vi "Drive Controller.vi"(8 "error in":errorcluster) -> ()   [LabVIEW 2015]
doc: "This VI executes continuously carrying out the current operation and responding to updates or new operation requests. It will often contain the timing or control code that is difficult to place directly in TeleOp. This VI generally opens all sensors and motors and isolates the rest of the robot code from knowing implementation details of how the operations are carried out."
uses:
  Drive Setpoints.ctl
  Drive Operations.ctl
  <vilib>/Rock Robotics/WPI/SafetyOutput/WPI_SafetyOutputConfigMenu.ctl
  <vilib>/Rock Robotics/WPI/CAN/TalonSRX/WPI_CANTalonSRX_APIControlMode.ctl
  <vilib>/Rock Robotics/WPI/CAN/TalonSRX/WPI_CANTalonSRX_APIFeedbackSelect.ctl
  <vilib>/Rock Robotics/WPI/MotorControl/WPI_MotorControlOpenCANTalonSRX.vi
  <vilib>/Rock Robotics/WPI/RobotDrive/WPI_RobotDriveOpen2MotorWithExistingMotors.vi
  Support Code/navX Library v2/navX Library v2.lvlib
panel:
  out "Setpoints":T1(graph)
  out "Current\nCmd":string
  # "Tip: It may be helpful to observe inputs and sensor values.\nYou may also want to display tuning or debugging controls."
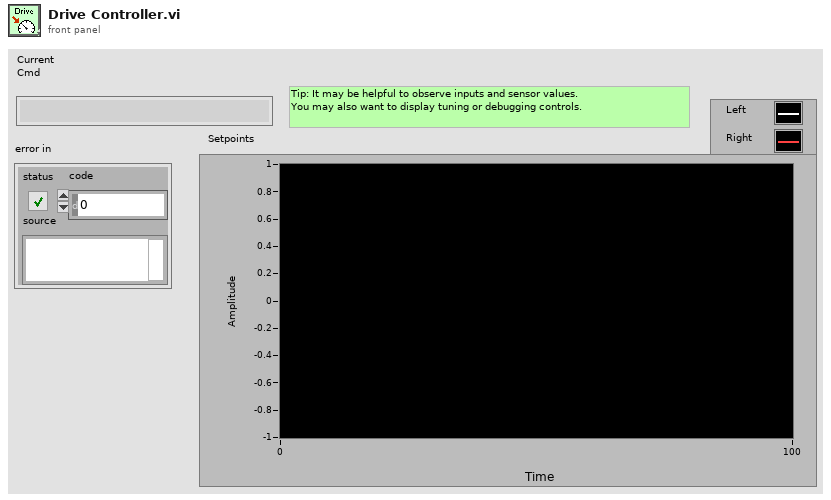
[diagram p1: front panel]
types:
  T1 = cluster{"Left Setpoint":dbl, "Right Setpoint":dbl}
  T2 = typedef "Drive Setpoints.ctl" = cluster{"Operation":T3, "Left Setpoint":dbl, "Right Setpoint":dbl, "Duration":dbl}
  T3 = typedef "Drive Operations.ctl" = enum16{"Reserve", "Read Current", "Immediate", "Drive for Time", "Drive for Distance"}
  T4 = typedef "WPI_SafetyOutputConfigMenu.ctl" = enum16{"Enable", "Disable"}
  T5 = typedef "WPI_CANTalonSRX_APIControlMode.ctl" = enum8{"Percent VBus", "Speed", "Position", "Slave", "Unchanged / Invalid", "Voltage Compensation", "Current", "Motion Profile"}
  T6 = typedef "WPI_CANTalonSRX_APIFeedbackSelect.ctl" = enum16{"Digital Quadrature Encoder", "Analog Potentiometer", "Analog Encoder", "Count on Quad-A (Rising-Edge)", "Count on Quad-A (Falling-Edge)", "CTR Magnetic Enc (Absolute)", "CTR Magnetic Enc (Relative)", "Pulse Width"}
  T7 = typedef "WPI_MotorControlDeviceRef.ctl" = cluster{"DeviceStatus":errorcluster, "Type":T8, "PWM":cluster{"PWM Channel":T9, "DeadBand":T10}, "CAN":cluster{"Device Number":u8, "Control Mode":T11, "Semaphore":T12, "Max Vout":dbl, "TalonSRX Control Mode":T5}, "Invert":bool}
  T8 = typedef "WPI_MotorControlType.ctl" = enum16{"PWM", "CAN", "CANTalonSRX"}
  T9 = typedef "FPGA_DIOPWMChannel.ctl" = enum8{"PWM 0", "PWM 1", "PWM 2", "PWM 3", "PWM 4", "PWM 5", "PWM 6", "PWM 7", "PWM 8", "PWM 9", "PWM MXP 0", "PWM MXP 1", "PWM MXP 2", "PWM MXP 3", "PWM MXP 4", "PWM MXP 5", "PWM MXP 6", "PWM MXP 7", "PWM MXP 8", "PWM MXP 9", "Invalid"}
  T10 = typedef "WPI_PWMDeadband.ctl" = cluster{"Name":string, "maxPositivePwm":i32, "minPositivePwm":i32, "centerPwm":i32, "maxNegativePwm":i32, "minNegativePwm":i32, "angularRange":u16}
  T11 = typedef "WPI_CANJaguar_ControlMode.ctl" = enum8{"Percent VBus", "Current", "Speed", "Position", "Voltage"}
  T12 = typedef "Semaphore RefNum" = refnum<k1>
  T13 = typedef "WPI_RobotDriveDevRef.ctl" = cluster{"DevStatus":errorcluster, "Motors[]":T7[], "Square Inputs":bool, "Max Output":dbl}
  T14 = typedef "navX Library v2.lvlib/Z900_navX_DeviceTypeDef.ctl" = cluster{"Interface":cluster{"Protocol":T15, "Update Rate (4Hz-60Hz)":u8, "navX Open TypeDef":variant}, "Notify Packet":refnum<notifier>, "Loop VI Refnum":refnum<vi>, "Ready to Close Occurrence Refnum":refnum<k4>}
  T15 = typedef "navX Library v2.lvlib/Z900_navX_ProtocolTypeDef.ctl" = enum16{"SERIAL", "I2C", "SPI"}
  T16 = typedef "Command Status Info.ctl" = cluster{"Name":string, "Status":T17, "notifier out":T18}
  T17 = typedef "Completion Status.ctl" = enum16{"Successful", "Aborted", "Incomplete"}
  T18 = typedef "Completion Notifier.ctl" = refnum<notifier>
  T19 = cluster{"SubSystem Data":T2, cluster{"Start Time (ms)":u32, "Iterations":i32}, cluster{"Command Info":T16, "Description":string, "SubSystem Data":T2, "notifier out":refnum<notifier>, "Subsystem Name":string}}
  T20 = cluster{"Yaw":dbl, "Roll":dbl, "Pitch":dbl, "Heading":dbl, "Fused Heading":dbl}
  T21 = typedef "WPI_CANTalonSRX_GlobalStatus.ctl" = cluster{"Applied Throttle":dbl, "Module Enabled":bool, "CAN Error":errorcluster, "Closed Loop Error":dbl, "Forward Limit Switch Closed":bool, "Reverse Limit Switch Closed":bool, "Sensor Position":dbl, "Sensor Velocity":dbl, "Current":dbl, "Sticky Fault - Over Temp":bool, "Sticky Fault - Under Voltage":bool, "Sticky Fault - Forward Limit":bool, "Sticky Fault - Reverse Limit":bool, "Sticky Fault - Forward Soft Limit":bool, "Sticky Fault - Reverse Soft Limit":bool, "Brake is Enabled":bool, "Encoder Position":dbl, "Encoder Velocity":dbl, "Encoder Index Count":dbl, "Encoder A Pin State":bool, "Encoder B Pin State":bool, "Encoder Index Pin State":bool, "Analog In":dbl, "Analog In Velocity":dbl, "Temperature (C)":dbl, "Battery Voltage":dbl, "Control 5 Is Supported":bool, "Current Profile Slot Select":dbl, "Pos Div 8":bool, "Vel Div 4":bool, "Pulse Width Position":i32, "Pulse Width Velocity":i32, "Pulse Width Rise To Rise (us)":i32, "Pulse Width Rise To Fall (us)":i32, "Mot Prof Active Is Under Run":bool, "Mot Prof Active Has Under Run":bool, "Mot Prof Active Is Last":bool, "Mot Prof Active Velocity Only":bool, "Mot Prof Active Is Valid":bool, "Mot Prof Buffer Is Full":bool, "Mot Prof Active Profile Slot Select":i32, "Mot Prof NextID":i32, "Mot Prof Count":i32, "Mot Prof Active Velocity":dbl, "Mot Prof Active Position":dbl, "Mot Prof Output Enable":i32}
  T22 = cluster{"Don't move motors while reserved":dbl, "Don't move motors while reserved":dbl}
  T23 = cluster{"SubSystem Data":T2, cluster{"Start Time (ms)":u32, "Iterations":i32}, "Default Command Arguments":cluster{"Command Info":T16, "Description":string, "SubSystem Data":T2, "notifier out":refnum<notifier>, "Subsystem Name":string}}
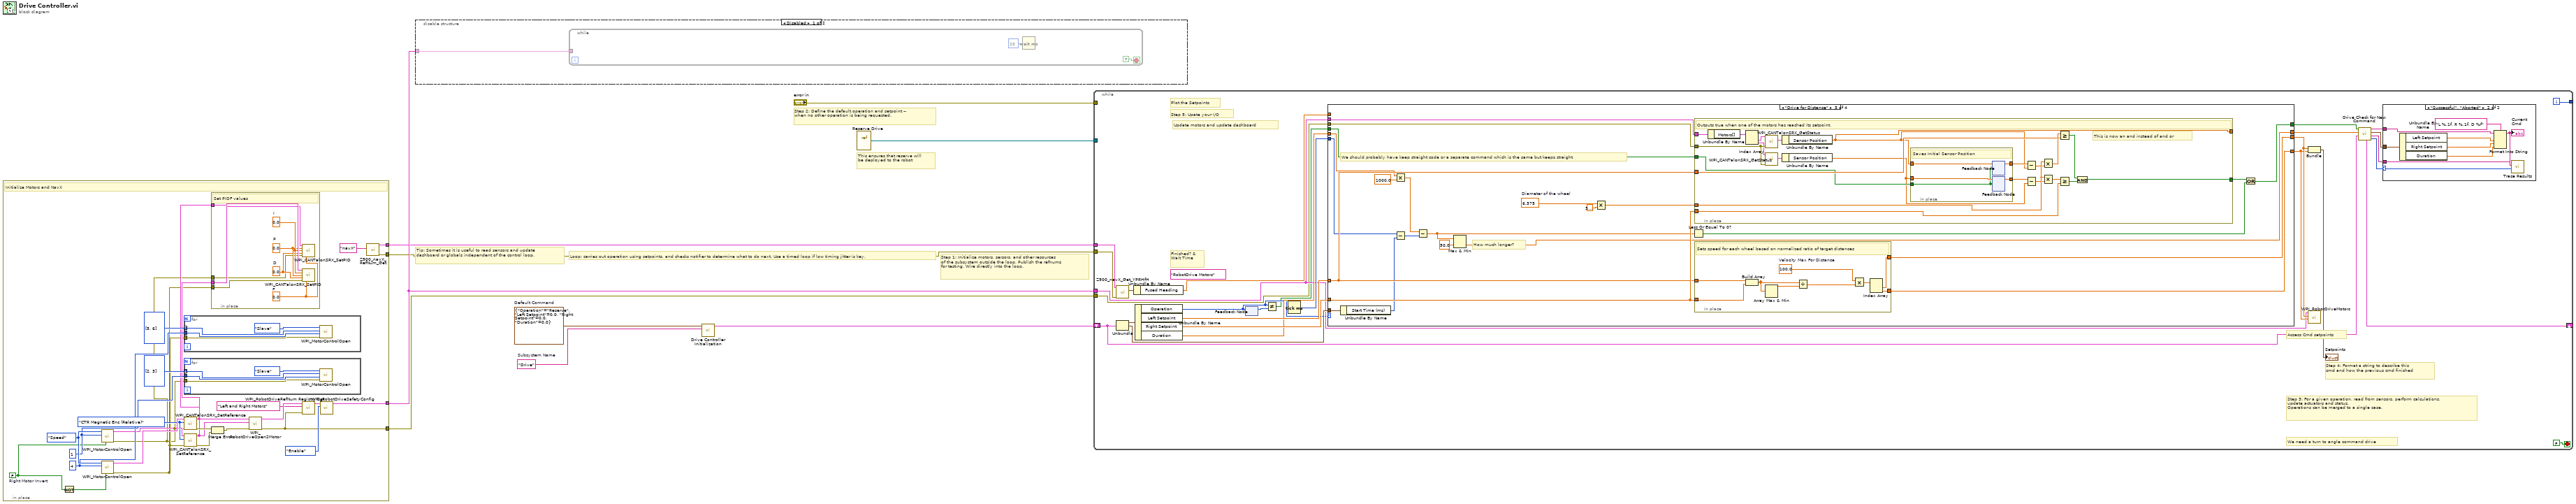
[diagram p0: block diagram]
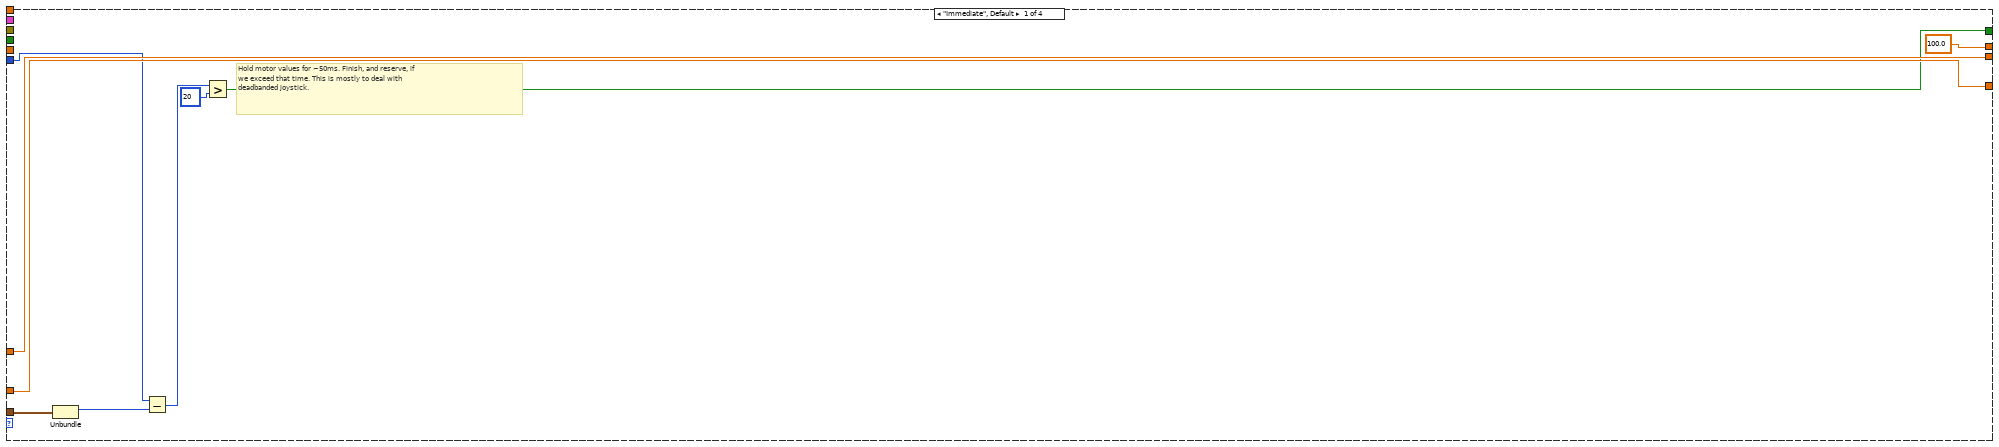
[diagram p4: hidden frame]
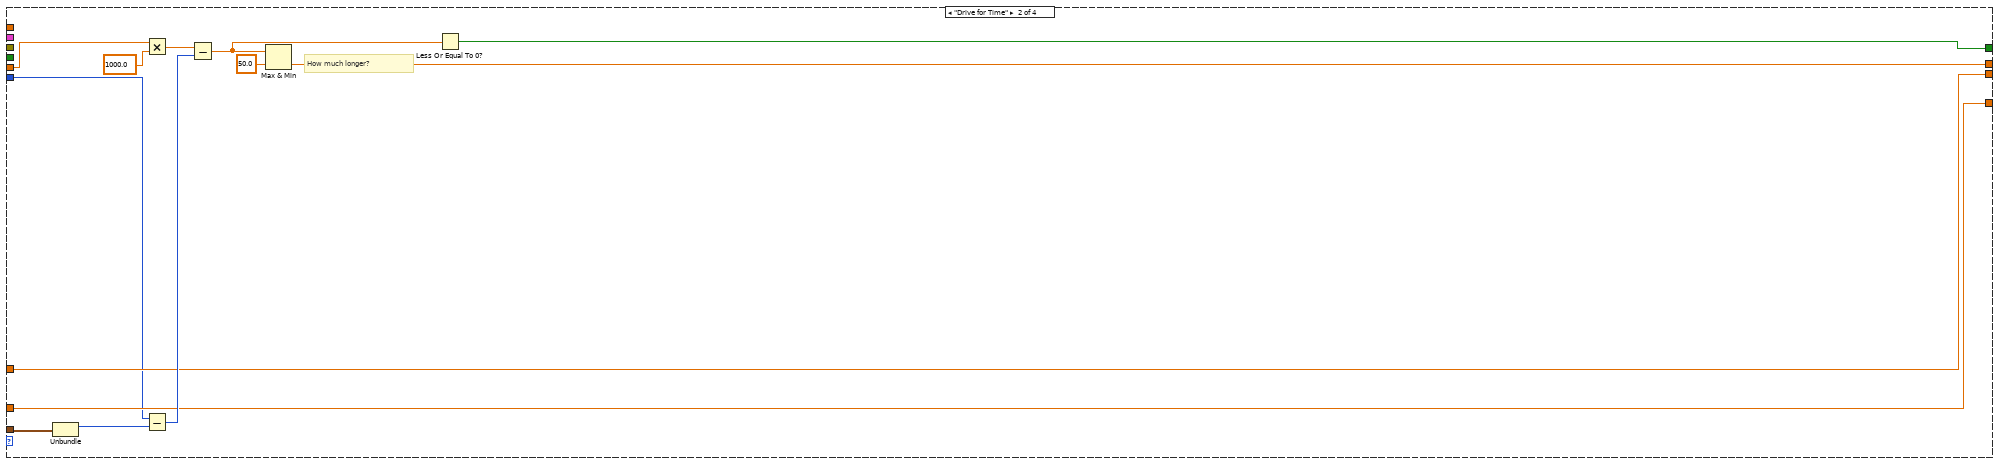
[diagram p5: hidden frame]
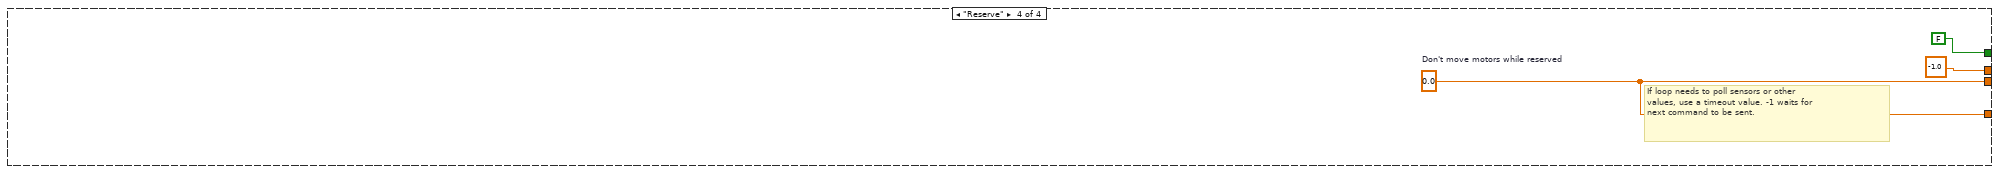
[diagram p6: hidden frame]
diagram:
  w8 = T2 {"Operation"=enum."Reserve", "Left Setpoint"=0.0, "Right Setpoint"=0.0, "Duration"=0.0}  # Default Command
  w9 = "Drive"  # Subsystem Name
  # "This ensures that reserve will\nbe deployed to the robot"
  # "Tip: Sometimes it is useful to read sensors and update\ndashboard or globals independent of the control loop."
  # "Step 2: Define the default operation and setpoint --\nwhen no other operation is being requested."
  # "Step 1: Initialize motors, sersors, and other resources\nof the subsystem outside the loop. Publish the refnums\nfor testing. Wire directly into the loop."
  # "Loop: carries out operation using setpoints, and checks notifier to determine what to do next. Use a timed loop if low timing jitter is key."
  n1 = in-place {
    in-place-border: [w31] -> w7
    in-place-border: [w17] -> w3
    in-place-border: [w11] -> w2
    in-place-border: [w10] -> w1
    w18 = WPI_CANTalonSRX_APIFeedbackSelect."CTR Magnetic Enc (Relative)" ("Feedback Reference")
    w25 = FALSE  # Right Motor Invert
    w28 = u8 4 ("Device Number")
    w29 = u8 1 ("Device Number")
    w30 = WPI_CANTalonSRX_APIControlMode."Speed" ("Control Mode")
    # "Initialize Motors and NavX"
    n2 = Not(x=w25) -> (.not. x?=w24:bool)
    n3 = call-poly <vilib>:"WPI_MotorControlOpen.vi"("Invert"=w25, "Device Number"=w29, "Control Mode"=w30) -> ("error out"=w13:errorcluster, "MotorControlDeviceRef"=w22:T7)  [unwired: 7 in]
    n4 = call-poly <vilib>:"WPI_MotorControlOpen.vi"("Invert"=w24, "Device Number"=w28, "Control Mode"=w30) -> ("error out"=w14:errorcluster, "MotorControlDeviceRef"=w23:T7)  [unwired: 7 in]
    n5 = for {
      tunnel: w28 -> [w47]
      tunnel: u8[] [5, 6] -> [w45] mode=indexing
      tunnel: w14 -> [w44]
      n6 = call-poly <vilib>:"WPI_MotorControlOpen.vi"("error in (no error)"=w44, "Master Device Number"=w47, "Device Number"=w45, "Control Mode"=WPI_CANTalonSRX_APIControlMode."Slave") -> ()  [unwired: 6 in, 2 out]
    }
    n7 = for {
      tunnel: w29 -> [w51]
      tunnel: u8[] [2, 3] -> [w49] mode=indexing
      tunnel: w13 -> [w48]
      n8 = call-poly <vilib>:"WPI_MotorControlOpen.vi"("error in (no error)"=w48, "Master Device Number"=w51, "Device Number"=w49, "Control Mode"=WPI_CANTalonSRX_APIControlMode."Slave") -> ()  [unwired: 6 in, 2 out]
    }
    n9 = call <vilib>:"WPI_CANTalonSRX_SetReference.vi"("error in (no error)"=w13, "Feedback Reference"=w18, "CAN Talon SRX Ref"=w23) -> ("error out"=w21:errorcluster, "CAN Talon SRX Ref"=w16:T7)  [unwired: 7 in]
    n10 = call <vilib>:"WPI_CANTalonSRX_SetReference.vi"("error in (no error)"=w14, "Feedback Reference"=w18, "CAN Talon SRX Ref"=w22) -> ("error out"=w20:errorcluster, "CAN Talon SRX Ref"=w15:T7)  [unwired: 7 in]
    n11 = in-place {
      in-place-border: w16 -> [w43]
      in-place-border: w15 -> [w42]
      in-place-border: w14 -> [w37]
      in-place-border: w13 -> [w36]
      w38 = 0.0  # F
      w39 = 0.0  # D
      w41 = 0.0  # I
      w40 = 0.0  # P
      # "Set PIDF values"
      n12 = call <vilib>:"WPI_CANTalonSRX_SetPID.vi"("CAN Talon SRX Ref"=w42, "P"=w40, "I"=w41, "D"=w39, "error in (no error)"=w36, "F"=w38) -> ()  [unwired: 8 in, 2 out]
      n13 = call <vilib>:"WPI_CANTalonSRX_SetPID.vi"("CAN Talon SRX Ref"=w43, "P"=w41, "I"=w40, "D"=w39, "error in (no error)"=w37, "F"=w38) -> ()  [unwired: 8 in, 2 out]
    }
    n14 = Merge Errors(w21, w20) -> (w19:errorcluster)
    n15 = call-poly <vilib>:"WPI_RobotDriveOpen2Motor.vi"("error in (no error)"=w19, "Right Motor Dev Ref"=w15, "Left Motor Dev Ref"=w16) -> ("error out"=w17:errorcluster, "RobotDriveDevRef"=w35:T13)  [unwired: 2 in, 5 out]
    n16 = call <vilib>:"WPI_RobotDriveRefNum Registry Set.vi"("error in (no error)"=w17, "refnum name"="Left and Right Motors", "RobotDriveDevRef"=w35) -> ("RobotDriveDevRef"=w33:T13)  [unwired: 1 in, 7 out]
    n17 = call <vilib>:"WPI_RobotDriveSafetyConfig.vi"("mode"=WPI_SafetyOutputConfigMenu."Enable", "RobotDriveDevRef"=w33) -> ("RobotDriveDevRef"=w31:T13)  [unwired: 8 in, 1 out]
    n18 = call "Z900_navX_RefNum_Get.vi"("refnum name"="navX") -> ("error out"=w10:errorcluster, "navX Device"=w11:T14)  [unwired: 9 in]
  }
  n19 = disable-structure shown="Disabled" {
    disable-tunnel: w7 -> [w52 _]
    frame Disabled {
      n20 = while {
        tunnel: w52 -> [_]
        stop <- FALSE stop-if-true
        n21 = Wait (ms)(milliseconds to wait=u32 20) -> ()  [unwired: 1 out]
      }
    }
    frame Enabled {
    }
  }
  n22 = call "Drive Controller Initialization.vi"("Subsystem Name"=w9, "Default Command"=w8) -> ("output cluster"=w5:T19)  [unwired: 9 in]
  n23 = vi-ref "Reserve Drive.vi"() -> (w4:refnum<vi>)
  n24 = while {
    shift-right: [w71] -> _
    shift-left: w5 -> [w64]
    tunnel: [w81] -> _
    tunnel: w7 -> [w63]
    tunnel: "error in" -> [_]
    tunnel: w4 -> [_]
    tunnel: w3 -> [w62]
    tunnel: w2 -> [w61]
    tunnel: w1 -> [w60]
    i -> [w81]
    stop <- FALSE stop-if-true
    (unwired) "RobotDrive Motors" ("Name")
    # "We need a turn to angle command drive"
    # "Step 5: Upate your I/O"
    # "Step 4: Format a string to describe this\ncmd and how the previous cmd finished"
    # "Update motors and update dashboard"
    # "Plot the Setpoints"
    # "Access Cmd setpoints"
    # "Finished? &\nWait Time"
    # "Step 3: For a given operation, read from sensors, perform calculations,\nupdate actuators and status.\nOperations can be merged to a single case."
    n25 = call "Z900_navX_Get_YPRHfH.vi"("error in (no error)"=w60, "navX Device"=w61) -> ("YRPHfH"=w59:T20)  [unwired: 6 in, 3 out]
    n26 = Unbundle(w64) -> ("SubSystem Data"=w77:T2, w65:cluster{"Start Time (ms)":u32, "Iterations":i32})  [unwired: 1 out]
    n27 = Unbundle By Name(w59) -> ("Fused Heading"=w55:dbl)
    n28 = Unbundle By Name(w77) -> ("Operation"=w57:T3, "Left Setpoint"=w76:dbl, "Right Setpoint"=w75:dbl, "Duration"=w74:dbl)
    n29 = feedback-in #1(w57) -> ()
    n30 = feedback #1() -> (w58:T3)  [unwired: 1 in]
    n31 = Not Equal?(x=w57, y=w58) -> (x != y?=w56:bool)
    n32 = Tick Count (ms)() -> (millisecond timer value=w73:u32)
    n33 = case shown="\"Drive for Distance\"" w57 {
      tunnel: [100.0 w102 w121 -1.0] -> w70
      tunnel: [w93 w108 w115 FALSE ("ignore previous (F)")] -> w69
      tunnel: w65 -> [w92 w110 w119 _]
      tunnel: [w99 w107 w129 w173] -> w79
      tunnel: [w98 w106 w136 w173] -> w78
      tunnel: w76 -> [w99 w107 w130 _]
      tunnel: w75 -> [w98 w106 w134 _]
      tunnel: w74 -> [_ w105 w120 _]
      tunnel: w73 -> [w94 w101 w117 _]
      tunnel: w63 -> [_ _ w133 _]
      tunnel: w62 -> [_ _ w135 _]
      tunnel: w56 -> [_ _ w127 _]
      tunnel: w55 -> [_ _ _ _]
      frame "Immediate", Default {
        # "Hold motor values for ~50ms. Finish, and reserve, if\nwe exceed that time. This is mostly to deal with\ndeadbanded joystick."
        n34 = Unbundle(w92) -> ("Start Time (ms)"=w95:u32)  [unwired: 1 out]
        n35 = Subtract(x=w94, y=w95) -> (x-y=w96:u32)
        n36 = Greater?(x=w96, y=u8 20 ("Left Motor")) -> (0:w93:bool)
      }
      frame "Drive for Time" {
        # "How much longer?"
        n37 = Unbundle(w110) -> ("Start Time (ms)"=w109:u32)  [unwired: 1 out]
        n38 = Multiply(x=w105, y=1000.0) -> (x*y=w112:dbl)
        n39 = Subtract(x=w101, y=w109) -> (x-y=w113:u32)
        n40 = Subtract(x=w112, y=w113) -> (x-y=w104:dbl)
        n41 = Max & Min(x=w104, y=50.0) -> (min(x,y)=w102:dbl)  [unwired: 1 out]
        n42 = Less Or Equal To 0?(x=w104) -> (x <= 0?=w108:bool)
      }
      frame "Drive for Distance" {
        w131 = 6.375  # Diameter of the wheel
        # "How much longer?"
        # "We should probably have keep straight code or a separate command which is the same but keeps straight"
        n43 = Unbundle By Name(w119) -> ("Start Time (ms)"=w118:u32)
        n44 = Multiply(x=w120, y=1000.0) -> (x*y=w125:dbl)
        n45 = Subtract(x=w117, y=w118) -> (x-y=w126:u32)
        n46 = Subtract(x=w125, y=w126) -> (x-y=w123:dbl)
        n47 = Max & Min(x=w123, y=50.0) -> (min(x,y)=w121:dbl)  [unwired: 1 out]
        n48 = Multiply(x=w131, y=3.141592653589793) -> (x*y=w128:dbl)
        n49 = Less Or Equal To 0?(x=w123) -> (x <= 0?=w114:bool)
        n50 = in-place {
          in-place-border: w130 -> [w167]
          in-place-border: w135 -> [w166]
          in-place-border: w134 -> [w165]
          in-place-border: w133 -> [w161]
          in-place-border: [w156] -> w116
          in-place-border: w128 -> [w153]
          in-place-border: [w149] -> _
          in-place-border: w127 -> [w152]
          # "This is now an and instead of and or"
          # "Outputs true when one of the motors has reached its setpoint."
          n51 = Unbundle By Name(w161) -> ("Motors[]"=w162:T7[])
          n52 = Index Array(array=w162) -> (element #1=w164:T7, element #2=w163:T7)  [unwired: 2 in]
          n53 = call <vilib>:"WPI_CANTalonSRX_GetStatus.vi"("error in (no error)"=w166, "CAN Talon SRX Ref"=w164) -> ("Talon SRX Status"=w155:T21)  [unwired: 7 in, 2 out]
          n54 = call <vilib>:"WPI_CANTalonSRX_GetStatus.vi"("error in (no error)"=w166, "CAN Talon SRX Ref"=w163) -> ("Talon SRX Status"=w154:T21)  [unwired: 7 in, 2 out]
          n55 = Unbundle By Name(w155) -> ("Sensor Position"=w149:dbl)
          n56 = Unbundle By Name(w154) -> ("Sensor Position"=w148:dbl)
          n57 = in-place {
            in-place-border: w149 -> [w172]
            in-place-border: w148 -> [w171]
            in-place-border: w152 -> [w170]
            in-place-border: [w169] -> w151
            in-place-border: [w168] -> w150
            # "Saves Initial Sensor Position"
            n58 = feedback #2() -> (w169:dbl)  [unwired: 1 in]
            n59 = feedback-in #2(w172, w170) -> ()
            n60 = feedback #3() -> (w168:dbl)  [unwired: 1 in]
            n61 = feedback-in #3(w171, w170) -> ()
          }
          n62 = Subtract(x=w151, y=w149) -> (x-y=w147:dbl)
          n63 = Subtract(x=w150, y=w148) -> (x-y=w146:dbl)
          n64 = Multiply(x=w153, y=w147) -> (x*y=w159:dbl)
          n65 = Multiply(x=w153, y=w146) -> (x*y=w160:dbl)
          n66 = Greater Or Equal?(x=w159, y=w167) -> (x >= y?=w158:bool)
          n67 = Greater Or Equal?(x=w160, y=w165) -> (x >= y?=w157:bool)
          n68 = And(x=w158, y=w157) -> (x .and. y?=w156:bool)
        }
        n69 = in-place {
          in-place-border: [w143] -> w129
          in-place-border: [w139] -> w136
          in-place-border: w130 -> [w138]
          in-place-border: w134 -> [w137]
          w145 = 100.0  # Velocity Max For Distance
          # "Sets speed for each wheel based on normalized ratio of target distances"
          n70 = Build Array(w138, w137) -> (w141:dbl[])
          n71 = Array Max & Min(array=w141) -> (max value=w142:dbl)  [unwired: 3 out]
          n72 = Divide(x=w141, y=w142) -> (x/y=w140:dbl[])
          n73 = Multiply(x=w145, y=w140) -> (x*y=w144:dbl[])
          n74 = Index Array(array=w144) -> (element #1=w143:dbl, element #2=w139:dbl)  [unwired: 2 in]
        }
        n75 = Or(x=w116, y=w114) -> (x .or. y?=w115:bool)
      }
      frame "Reserve" {
        w173 = 0.0  # Don't move motors while reserved
        # "If loop needs to poll sensors or other\nvalues, use a timeout value. -1 waits for\nnext command to be sent."
      }
    }
    n76 = Bundle("Don't move motors while reserved"=w79, "Don't move motors while reserved"=w78) -> (→"Setpoints":T22)  [unwired: 1 in]
    n77 = call <vilib>:"WPI_RobotDriveMotors.vi"("RightSpeed"=w78, "LeftSpeed"=w79, "RobotDriveDevRef"=w63) -> ()  [unwired: 1 in, 8 out]
    n78 = call "Drive Check for New Command.vi"("input cluster"=w64, "Wait time (ms)"=w70, "Finished?"=w69) -> ("Completion"=w72:T17, "Subsystem Name"=w66:string, "SetPoint"=w67:T2, "Initial Trace String"=w68:string, "output cluster"=w71:T23)  [unwired: 4 in]
    n79 = case shown="\"Successful\", \"Aborted\"" w72 {
      selector: w72 -> [_ w91]
      tunnel: w68 -> [_ w86]
      tunnel: w67 -> [_ w87]
      tunnel: w66 -> [_ w83]
      frame "Incomplete", Default {
        # "Continuing current command"
      }
      frame "Successful", "Aborted" {
        # "Report and setup for next command"
        n80 = Unbundle By Name(w87) -> ("Left Setpoint"=w89:dbl, "Right Setpoint"=w90:dbl, "Duration"=w84:dbl)
        n81 = Format Into String(format string="L %.1f, R %.1f, D %f", initial string=w86, w89, w90, w84) -> (resulting string=w85:string)  [unwired: 1 in, 1 out]
        "Current\nCmd" <- w85
        n82 = call <vilib>:"Trace Results.vi"("Status of previous command"=w91, "Description"=w85, "Subsystem"=w83) -> ()  [unwired: 9 in]
      }
    }
  }
